vi "dfd_FXP Filtering Statistics.vi"(8 "filtering statistics in":T3(array[cluster]) {"statistics information"."min value" format="%.2f"; "statistics information"."max value" format="%.2f"; "Quantizer Source" items=["Coefficients a/k"=0, "Coefficients b/v"=7, "Input"=1, "Output"=2, "Multiplicand"=3, "Product"=4, "Sum"=5, "Delay"=6]}, 10 "source":T4=7 items=["Coef a/k"=0, "Coef b/v"=7, "Input"=1, "Output"=2, "Multiplicand"=3, "Product"=4, "Sum"=5, "Delay"=6, "Gain"=8], 11 "new data":T2={"max value"=-inf, "min value"=inf, "#overflows"=0, "#underflows"=0, "#operations"=1} {"min value" format="%.2f"; "max value" format="%.2f"}) -> (0 "filtering statistics out":T3(array[cluster]) {"statistics information"."min value" format="%.2f"; "statistics information"."max value" format="%.2f"; "Quantizer Source" items=["Coefficients a/k"=0, "Coefficients b/v"=7, "Input"=1, "Output"=2, "Multiplicand"=3, "Product"=4, "Sum"=5, "Delay"=6]})   [LabVIEW 2017, in "NI_DigFilter_FXP.lvlib"]
uses:
  <vilib>/addons/Digital Filter Design/NI_DigFilter_FXP.lvlib
  <vilib>/addons/Digital Filter Design/_Objects.llb/dfd_Internal Quantization Srcs.ctl
  <vilib>/addons/Digital Filter Design/_Objects.llb/DFD FXP Statistics Data.ctl
  <vilib>/addons/Digital Filter Design/_Objects.llb/DFD Quantization Sources.ctl
  <vilib>/addons/Digital Filter Design/NI_DigFilterLicensed.lvlib
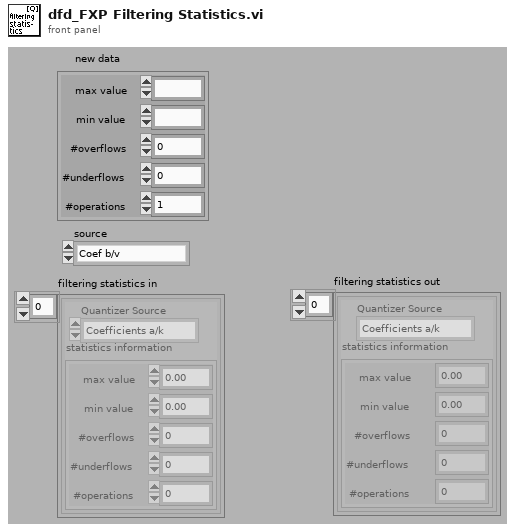
[diagram p1: front panel]
types:
  T1 = typedef "NI_DigFilterLicensed.lvlib/DFD Quantization Sources.ctl" = u16
  T2 = typedef "NI_DigFilterLicensed.lvlib/DFD FXP Statistics Data.ctl" = cluster{"max value":ext, "min value":ext, "#overflows":i32, "#underflows":i32, "#operations":i32}
  T3 = cluster{"Quantizer Source":T1, "statistics information":T2}[]
  T4 = typedef "NI_DigFilterLicensed.lvlib/dfd_Internal Quantization Srcs.ctl" = u16
  T5 = cluster{"Quantizer Source":T1, "statistics information":T2}
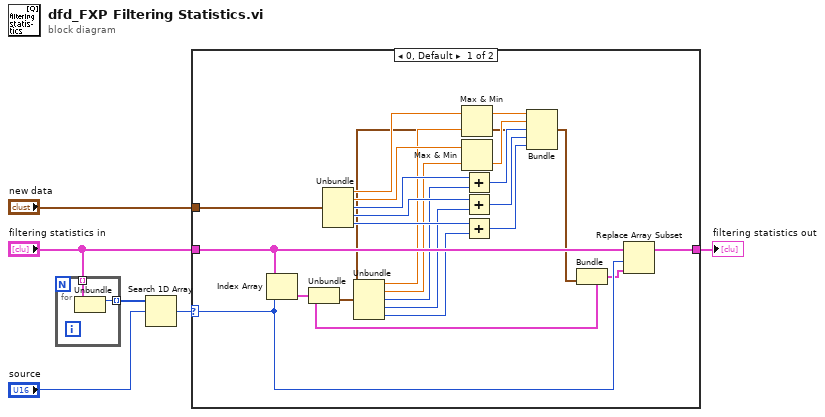
[diagram p0: block diagram]
diagram:
  n1 = for {
    tunnel: "filtering statistics in" -> [w8] mode=indexing
    tunnel: [w7] -> w3 mode=indexing
    n2 = Unbundle(w8) -> ("Quantizer Source"=w7:T1)  [unwired: 1 out]
  }
  n3 = Search 1D Array(1D array=w3, element="source") -> (index of element=w1:i32)  [unwired: 1 out]
  n4 = case shown="0, Default" w1 {
    selector: w1 -> [w28 _]
    tunnel: "new data" -> [w31 _]
    tunnel: [w30 w32] -> w5
    tunnel: "filtering statistics in" -> [w29 w32]
    frame 0, Default {
      n5 = Index Array(array=w29, index=w28) -> (element=w10:T5)
      n6 = Unbundle(w10) -> ("statistics information"=w9:T2)  [unwired: 1 out]
      n7 = Unbundle(w31) -> ("max value"=w27:ext, "min value"=w26:ext, "#overflows"=w25:i32, "#underflows"=w24:i32, "#operations"=w23:i32)
      n8 = Unbundle(w9) -> ("max value"=w22:ext, "min value"=w21:ext, "#overflows"=w20:i32, "#underflows"=w19:i32, "#operations"=w18:i32)
      n9 = Max & Min(x=w27, y=w22) -> (max(x,y)=w17:ext)  [unwired: 1 out]
      n10 = Max & Min(x=w26, y=w21) -> (min(x,y)=w16:ext)  [unwired: 1 out]
      n11 = Add(x=w25, y=w20) -> (x+y=w15:i32)
      n12 = Add(x=w24, y=w19) -> (x+y=w14:i32)
      n13 = Add(x=w23, y=w18) -> (x+y=w13:i32)
      n14 = Bundle(cluster=w9, "max value"=w17, "min value"=w16, "#overflows"=w15, "#underflows"=w14, "#operations"=w13) -> (w12:T2)
      n15 = Bundle(cluster=w10, "statistics information"=w12) -> (w11:T5)  [unwired: 1 out]
      n16 = Replace Array Subset(array=w29, new element=w11, index=w28) -> (w30:T3)
    }
    frame ..-1 {
    }
  }
  "filtering statistics out" <- w5
